vi "K_S30_VISA F31.vi"(4 "error in":errorcluster, 5 "Coeff. Nr.":u8=64, 6 "Coeff":sgl format="%.6e", 7 "Address":u8=250) -> (0 "error out":errorcluster)   [LabVIEW 2012]
panel:
  # "Function 31: Write coefficient\nV1.0, b.v."
  # "Note: With that function you write coefficients!!"
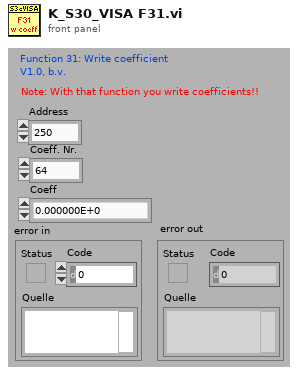
[diagram p1: front panel]
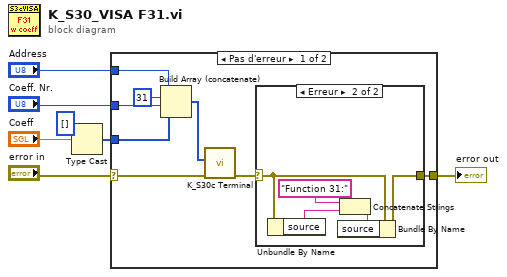
[diagram p0: block diagram]
diagram:
  n1 = Type Cast(type=u8[] [] ("response"), x="Coeff") -> (*(type *) &x=w1:u8[])
  n2 = case shown="Pas d'erreur" "error in" {
    selector: "error in" -> [w12 w22]
    tunnel: "Address" -> [w15 _]
    tunnel: [w10 w22] -> w5
    tunnel: "Coeff. Nr." -> [w9 _]
    tunnel: w1 -> [w8 _]
    frame No Error {
      n3 = Build Array (concatenate)(w15, u8 31 ("Element"), w9, w8) -> (w13:u8[])
      n4 = call "K_S30c Terminal.vi"("error in"=w12, "request"=w13) -> ("error out"=w11:errorcluster)  [unwired: 4 in, 1 out]
      n5 = case shown="Erreur" w11 {
        selector: w11 -> [w16 w21]
        tunnel: [w16 w19] -> w10
        frame No Error {
        }
        frame Error {
          n6 = Unbundle By Name(w21) -> ("source"=w18:string)
          n7 = Concatenate Strings("Function 31:" ("String"), w18) -> (w20:string)
          n8 = Bundle By Name(cluster=w21, "source"=w20) -> (w19:errorcluster)
        }
      }
    }
    frame Error {
    }
  }
  "error out" <- w5
